vi "get unit string.vi"(8 "error in (no error)":errorcluster, 11 "Variant":variant) -> (0 "error out":errorcluster, 3 "String":string)   [LabVIEW 2017, in "DSF Data Viewer.lvlib"]
uses:
  DSF Data Viewer.lvlib
  <vilib>/Utility/Data Type/NI_Data Type.lvlib
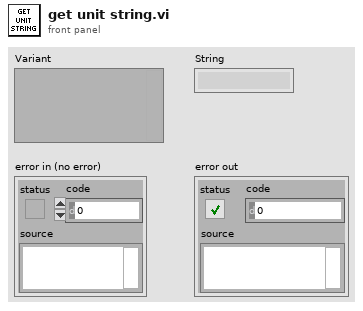
[diagram p1: front panel]
types:
  T1 = typedef "NI_Data Type.lvlib/Unit Info.ctl" = cluster{"Unit Type":T2, "Exponent":i16}
  T2 = typedef "NI_Data Type.lvlib/Unit Type.ctl" = enum16{"Radians", "Steradians", "Seconds", "Meters", "Kilograms", "Amperes", "Kelvins", "Moles", "Candelas", "InvalidUnit"}
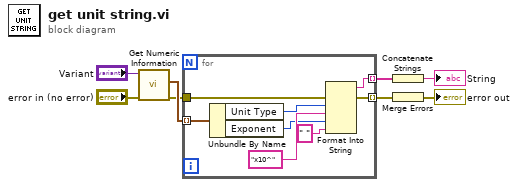
[diagram p0: block diagram]
diagram:
  n1 = call <vilib>:"Get Numeric Information.vi"("error in (no error)"="error in (no error)", "Variant"="Variant") -> ("error out"=w3:errorcluster, "Units"=w5:T1[])  [unwired: 6 in, 2 out]
  n2 = for {
    tunnel: w5 -> [w16] mode=indexing
    tunnel: [w12] -> w7 mode=indexing
    tunnel: w3 -> [w10]
    tunnel: [w9] -> w2 mode=indexing
    n3 = Unbundle By Name(w16) -> ("Unit Type"=w15:T2, "Exponent"=w13:i16)
    n4 = Format Into String(error in=w10, w15, "x10^" ("initial string"), w13, " " ("initial string")) -> (resulting string=w12:string, error out=w9:errorcluster)  [unwired: 2 in]
  }
  n5 = Concatenate Strings(w7) -> (→"String":string)
  n6 = Merge Errors(w2) -> (→"error out":errorcluster)
